vi "Match tag img Ascii and Unicode.vi"(0 "Type and run direction":T1=enum."ASCII", 7 "String":string, 11 "error in (no error)":errorcluster) -> (8 "Text [ ]":cluster{"ASCII":string, "Image?":bool}[](array[cluster]), 15 "error out":errorcluster)   [LabVIEW 2019]
doc: "Version 2.0\nDeveloped by Jean-Marc Simard\nCopyright © 2010, Exaprom Inc.\nAll rights reserved.\nLicense: BSD"
uses:
  <userlib>/Exaprom PDF/Controls/Text Controls/Unicode/Type and run direction.ctl
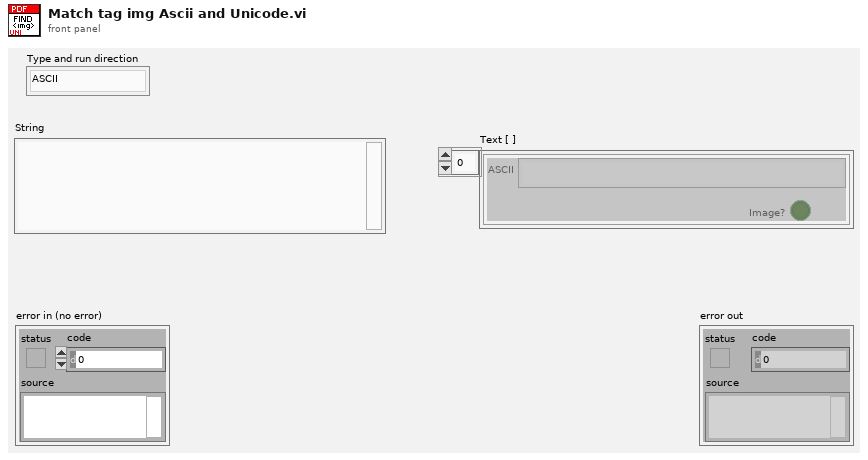
[diagram p1: front panel]
types:
  T1 = typedef "Type and run direction.ctl" = enum16{"Select", "ASCII", "UTF-16", "UTF-16 (default)", "UTF-16 (LTR)", "UTF-16 (RTL)"}
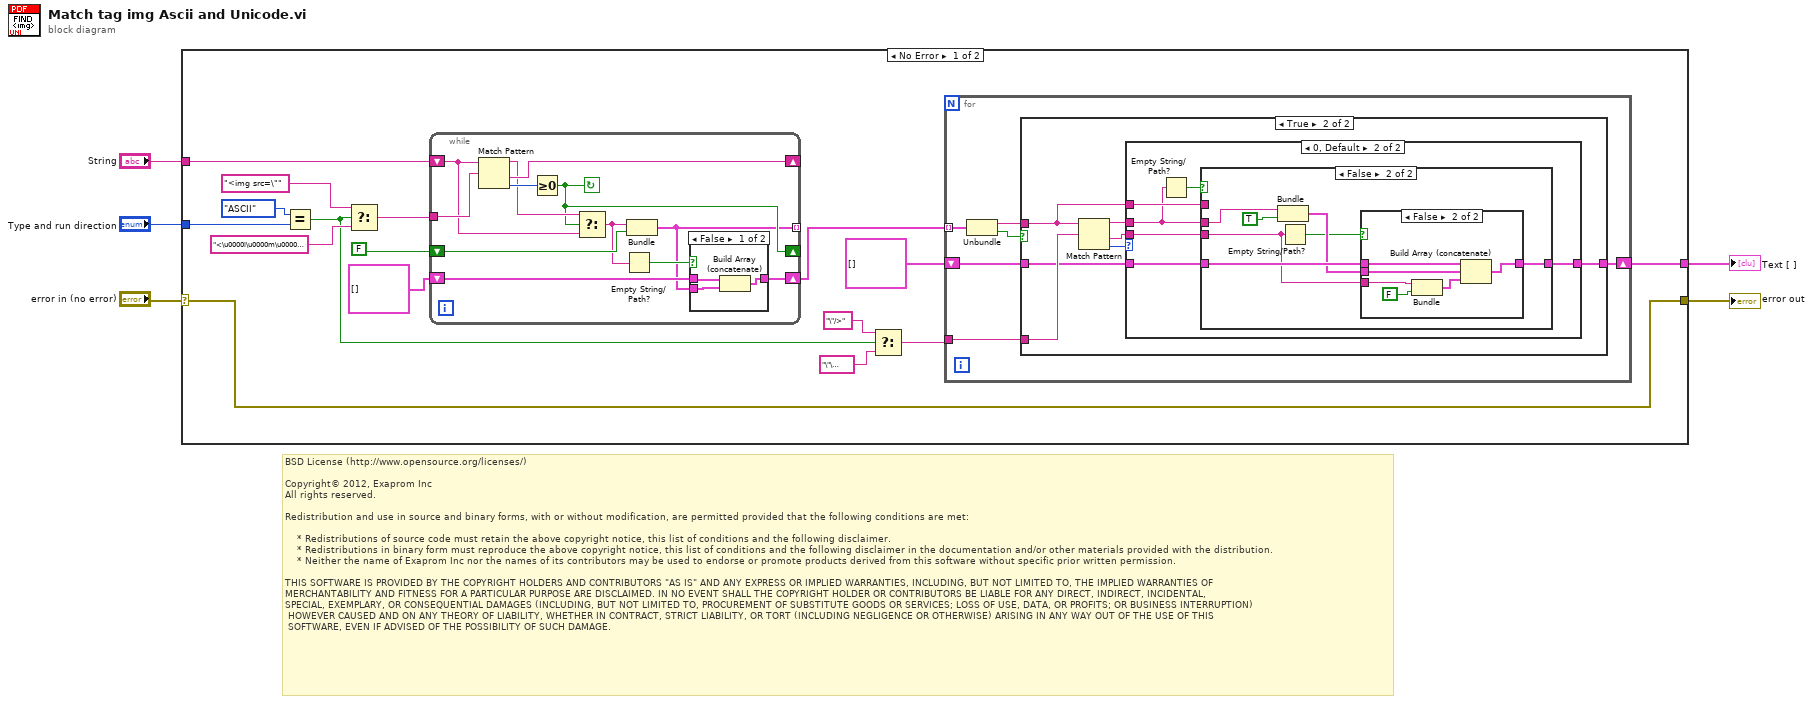
[diagram p0: block diagram]
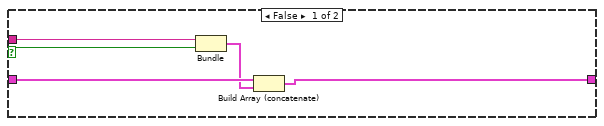
[diagram p2: hidden frame]
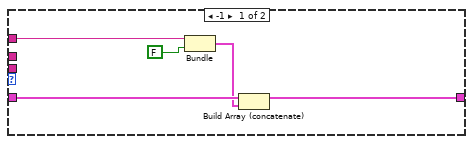
[diagram p3: hidden frame]
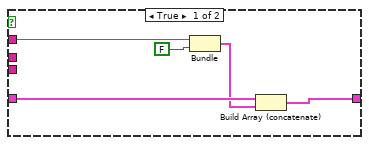
[diagram p4: hidden frame]
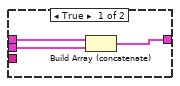
[diagram p5: hidden frame]
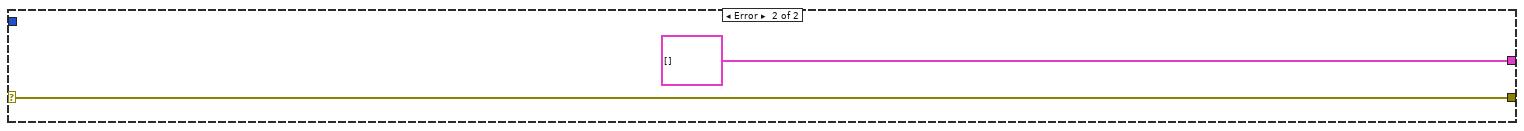
[diagram p7: hidden frame]
diagram:
  # "BSD License (http://www.opensource.org/licenses/)\n\nCopyright© 2012, Exaprom Inc\nAll rights reserved.\n\nRedistribution and use in source and binary forms, with or without modification, are permitted provided that the following conditions are met:\n\n    * Redistributions of source code must retain the above copyright notice, this list of conditions and the following disclaimer.\n    * Redistributions in binary form must reproduce the above copyright notice, this list of conditions and the following disclaimer in the documentation and/or other materials provided with the distribution.\n    * Neither the name of Exaprom Inc nor the names of its contributors may be used to endorse or promote products derived from this software without specific prior written permission.\n\nTHIS SOFTWARE IS PROVIDED BY THE COPYRIGHT HOLDERS AND CONTRIBUTORS \"AS IS\" AND ANY EXPRESS OR IMPLIED WARRANTIES, INCLUDING, BUT NOT LIMITED TO, THE IMPLIED WARRANTIES OF \nMERCHANTABILITY AND FITNESS FOR A PARTICULAR PURPOSE ARE DISCLAIMED. IN NO EVENT SHALL THE COPYRIGHT HOLDER OR CONTRIBUTORS BE LIABLE FOR ANY DIRECT, INDIRECT, INCIDENTAL,\nSPECIAL, EXEMPLARY, OR CONSEQUENTIAL DAMAGES (INCLUDING, BUT NOT LIMITED TO, PROCUREMENT OF SUBSTITUTE GOODS OR SERVICES; LOSS OF USE, DATA, OR PROFITS; OR BUSINESS INTERRUPTION)\n HOWEVER CAUSED AND ON ANY THEORY OF LIABILITY, WHETHER IN CONTRACT, STRICT LIABILITY, OR TORT (INCLUDING NEGLIGENCE OR OTHERWISE) ARISING IN ANY WAY OUT OF THE USE OF THIS\n SOFTWARE, EVEN IF ADVISED OF THE POSSIBILITY OF SUCH DAMAGE."
  n1 = case shown="No Error" "error in (no error)" {
    selector: "error in (no error)" -> [w20 w89]
    tunnel: "String" -> [w21 _]
    tunnel: [w20 w89] -> w4
    tunnel: "Type and run direction" -> [w16 _]
    tunnel: [w19 cluster{"ASCII":string, "Image?":bool}[] [] ("Array")] -> w1
    frame No Error {
      n2 = Equal?(x=Type_and_run_direction."ASCII" ("Type and run direction"), y=w16) -> (x = y?=w9:bool)
      n3 = Select(t="<img src=\"" ("regular expression"), s=w9, f="<\u0000i\u0000m\u0000g\u0000 \u0000s\u0000r\u0000c\u0000=\u0000\"\u0000" ("regular expression")) -> (s? t:f=w15:string)
      n4 = while {
        shift-right: [w81] -> _
        shift-left: w21 -> [w78]
        tunnel: w15 -> [w82]
        tunnel: [w72] -> _ mode=indexing
        shift-right: [w77] -> _
        shift-left: FALSE -> [w80]
        shift-right: [w73] -> w7
        shift-left: cluster{"String":string, bool}[] [] -> [w74]
        stop <- w77 continue-if-true
        n5 = Match Pattern(string=w78, regular expression=w82) -> (before substring=w79:string, after substring=w81:string, offset past match=w83:i32)  [unwired: 1 in, 1 out]
        n6 = Greater Or Equal To 0?(x=w83) -> (x >= 0?=w77:bool)
        n7 = Select(t=w79, s=w77, f=w78) -> (s? t:f=w75:string)
        n8 = Empty String/Path?(string/path=w75) -> (empty?=w76:bool)
        n9 = Bundle("String"=w75, w80) -> (w72:cluster{"String":string, bool})  [unwired: 1 in]
        n10 = case shown="False" w76 {
          tunnel: w74 -> [w86 w87]
          tunnel: [w85 w87] -> w73
          tunnel: w72 -> [w84 _]
          frame False {
            n11 = Build Array (concatenate)(w86, w84) -> (w85:cluster{"String":string, bool}[])
          }
          frame True {
          }
        }
      }
      n12 = Select(t="\"/>", s=w9, f="\"\u0000/\u0000>\u0000") -> (s? t:f=w10:string)
      n13 = for {
        tunnel: w7 -> [w27] mode=indexing
        tunnel: w10 -> [w22]
        shift-right: [w23] -> w19
        shift-left: cluster{"ASCII":string, "Image?":bool}[] [] ("Array") -> [w24]
        n14 = Unbundle(w27) -> ("String"=w25:string, w26:bool)
        n15 = case shown="True" w26 {
          selector: w26 -> [w28 _]
          tunnel: w25 -> [w32 w35]
          tunnel: w22 -> [_ w39]
          tunnel: w24 -> [w31 w34]
          tunnel: [w29 w33] -> w23
          frame False {
            n16 = Bundle("String"=w32, w28) -> (w30:cluster{"String":string, bool})  [unwired: 1 in]
            n17 = Build Array (concatenate)(w31, w30) -> (w29:cluster{"String":string, "Image?":bool}[])
          }
          frame True {
            n18 = Match Pattern(string=w35, regular expression=w39) -> (before substring=w37:string, after substring=w36:string, offset past match=w38:i32)  [unwired: 1 in, 1 out]
            n19 = case shown="0, Default" w38 {
              tunnel: w37 -> [_ w48]
              tunnel: w36 -> [_ w47]
              tunnel: w35 -> [w44 w49]
              tunnel: w34 -> [w43 w46]
              tunnel: [w42 w45] -> w33
              frame -1 {
                n20 = Bundle("String"=w44, FALSE) -> (w41:cluster{"String":string, bool})  [unwired: 1 in]
                n21 = Build Array (concatenate)(w43, w41) -> (w42:cluster{"String":string, "Image?":bool}[])
              }
              frame 0, Default {
                n22 = Empty String/Path?(string/path=w48) -> (empty?=w50:bool)
                n23 = case shown="False" w50 {
                  tunnel: w49 -> [w55 _]
                  tunnel: w48 -> [_ w59]
                  tunnel: w47 -> [_ w57]
                  tunnel: w46 -> [w54 w62]
                  tunnel: [w52 w60] -> w45
                  frame True {
                    n24 = Bundle("String"=w55, FALSE) -> (w53:cluster{"String":string, bool})  [unwired: 1 in]
                    n25 = Build Array (concatenate)(w54, w53) -> (w52:cluster{"String":string, "Image?":bool}[])
                  }
                  frame False {
                    n26 = Bundle("String"=w59, TRUE) -> (w61:cluster{"String":string, bool})  [unwired: 1 in]
                    n27 = Empty String/Path?(string/path=w57) -> (empty?=w58:bool)
                    n28 = case shown="False" w58 {
                      tunnel: w62 -> [w65 w71]
                      tunnel: w61 -> [w64 w70]
                      tunnel: [w63 w69] -> w60
                      tunnel: w57 -> [_ w68]
                      frame True {
                        n29 = Build Array (concatenate)(w65, w64) -> (w63:cluster{"String":string, "Image?":bool}[])
                      }
                      frame False {
                        n30 = Bundle("String"=w68, FALSE) -> (w67:cluster{"String":string, bool})  [unwired: 1 in]
                        n31 = Build Array (concatenate)(w71, w70, w67) -> (w69:cluster{"String":string, "Image?":bool}[])
                      }
                    }
                  }
                }
              }
            }
          }
        }
      }
    }
    frame Error {
    }
  }
  "error out" <- w4
  "Text [ ]" <- w1
